vi "SendBuffer.vi"(1 "销毁":bool) -> (0 "VCI_CAN_BUF_T":refnum<queue>)   [LabVIEW 2011]
uses:
  _USB_CAN_SEND_BUFF_UNIT_.ctl
panel:
  # "通信数据接收队列"
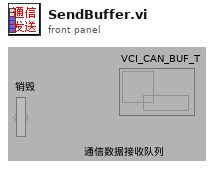
[diagram p1: front panel]
types:
  T1 = typedef "_USB_CAN_SEND_BUFF_UNIT_.ctl" = cluster{"datalen":u8, "data":u8[], "id":u8[], "extended":bool, "remote":bool}
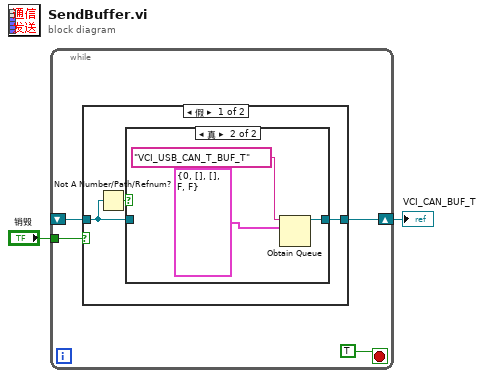
[diagram p0: block diagram]
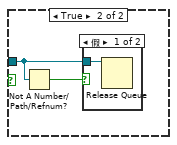
[diagram p3: hidden frame]
diagram:
  n1 = while {
    shift-right: [w4] -> w1
    shift-left: _ -> [w5]
    tunnel: "销毁" -> [w3]
    stop <- TRUE stop-if-true
    n2 = case shown="假" w3 {
      tunnel: w5 -> [w8 w14]
      tunnel: [w7 _] -> w4
      frame False {
        n3 = Not A Number/Path/Refnum?(number/path/refnum=w8) -> (NaN/Path/Refnum?=w9:bool)
        n4 = case shown="真" w9 {
          tunnel: w8 -> [w10 _]
          tunnel: [w10 w12] -> w7
          frame False {
          }
          frame True {
            n5 = Obtain Queue(name (unnamed)="VCI_USB_CAN_T_BUF_T" ("名称（未命名）"), element data type=T1 {"datalen"=0, "data"=[], "id"=[], "extended"=FALSE, "remote"=FALSE} ("VCI_CAN_BUF_T")) -> (queue out=w12:refnum<queue>)  [unwired: 3 in, 2 out]
          }
        }
      }
      frame True {
        n6 = Not A Number/Path/Refnum?(number/path/refnum=w14) -> (NaN/Path/Refnum?=w15:bool)
        n7 = case shown="假" w15 {
          tunnel: w14 -> [w16 _]
          frame False {
            n8 = Release Queue(queue=w16) -> ()  [unwired: 2 in, 3 out]
          }
          frame True {
          }
        }
      }
    }
  }
  "VCI_CAN_BUF_T" <- w1
